vi "Implement Authenticate.vi"(8 "error in (no error)":errorcluster, 10 "Challenge Dict":string, 11 "WampScramAuthenticator in":refnum<class "WampScramAuthenticator.lvclass">) -> (0 "error out":errorcluster, 1 "Authenticate Dict":string, 2 "Authenticate Signature":string, 3 "WampScramAuthenticator out":refnum<class "WampScramAuthenticator.lvclass">)   [LabVIEW 2020, in "wamplv.lvlib" / "WampScramAuthenticator.lvclass"]
uses:
  WampScramAuthenticator.lvclass
  TypeDefs/Authenticate Extra data.ctl
  efa46892-2042-4062-853f-90a4d9cfa7e0.vi
  1957a34c-6116-4582-936f-7ec411d64d2c.vi
  32660840-3418-4907-9075-9fb4615483c7.vi
  <vilib>/JDP Science/JSONtext/Variant to JSON Text.vi
  <vilib>/JDP Science/JSONtext/Set Item.vi
  <vilib>/JDP Science/JSONtext/LVClass Serializer/JSONtext LVClass Serializer.lvclass
  WampScramAuthenticator.lvclass/WampScramAuthenticator.ctl
  Utils/Utils.lvclass
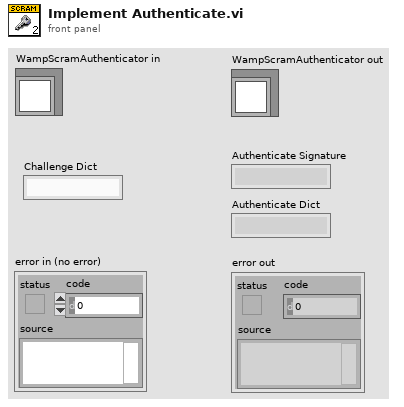
[diagram p1: front panel]
types:
  T1 = typedef "wamplv.lvlib/WampScramAuthenticator.lvclass/Challenge data.ctl" = cluster{"Nonce":string, "kdf":string, "HMAC parameters":T2}
  T2 = typedef "wamplv.lvlib/WampScramAuthenticator.lvclass/HMAC parameters.ctl" = cluster{"Salt":string, "Iterations":i32}
  T3 = typedef "wamplv.lvlib/WampScramAuthenticator.lvclass/Authenticate Extra data.ctl" = cluster{"Nonce":string, "channel_binding":string, "cbind_data":string}
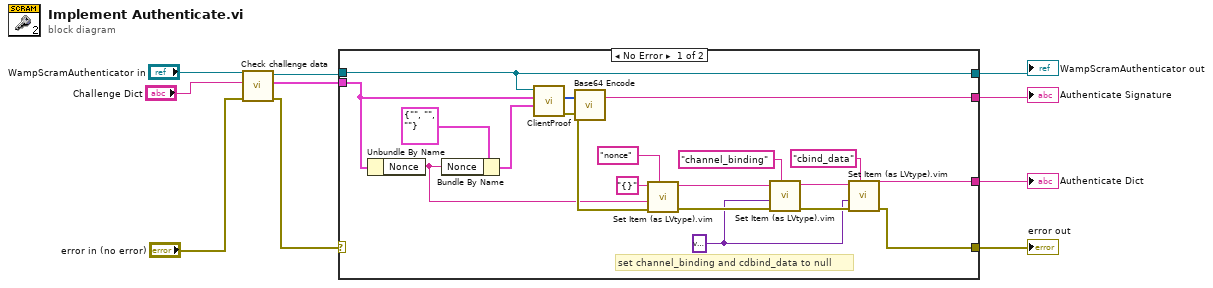
[diagram p0: block diagram]
diagram:
  n1 = call "Check challenge data.vi"("error in (no error)"="error in (no error)", "Challenge Dict"="Challenge Dict", "WampScramAuthenticator in"="WampScramAuthenticator in") -> ("error out"=w4:errorcluster, "Challene data"=w3:T1, "WampScramAuthenticator out"=w5:refnum<class "WampScramAuthenticator.lvclass">)  [unwired: 6 in]
  n2 = case shown="No Error" w4 {
    selector: w4 -> [_ w30]
    tunnel: w5 -> [w28 w31]
    tunnel: [w28 w31] -> w10
    tunnel: [w14 w30] -> w9
    tunnel: w3 -> [w27 _]
    tunnel: [w23 _] -> w2
    tunnel: [w12 _] -> w1
    frame No Error {
      w15 = variant
      # "set channel_binding and cdbind_data to null"
      n3 = Unbundle By Name(w27) -> ("Nonce"=w11:string)
      n4 = Bundle By Name(cluster=T3 {"Nonce"="", "channel_binding"="", "cbind_data"=""} ("Authenticate Extra Data"), "Nonce"=w11) -> (w22:T3)
      n5 = call "ClientProof.vi"("Authenticate Extra  Data"=w22, "Challenge data"=w27, "WampScramAuthenticator in"=w28) -> ("error out"=w13:errorcluster, "ClientProof"=w26:u8[])  [unwired: 6 in, 1 out]
      n6 = call "Base64 Encode.vi"("Bytes"=w26) -> ("Base64 sring out"=w23:string)  [unwired: 2 in]
      n7 = call "Set Item (as LVtype).vim"("$Path or Item Name"="nonce", "error in (no error)"=w13, "Anything"=w11, "JSON"="{}") -> ("error out"=w20:errorcluster, "<JSON>"=w21:string)  [unwired: 4 in, 1 out]
      n8 = call "Set Item (as LVtype).vim"("$Path or Item Name"="channel_binding", "error in (no error)"=w20, "Anything"=w15, "JSON"=w21) -> ("error out"=w17:errorcluster, "<JSON>"=w18:string)  [unwired: 4 in, 1 out]
      n9 = call "Set Item (as LVtype).vim"("$Path or Item Name"="cbind_data", "error in (no error)"=w17, "Anything"=w15, "JSON"=w18) -> ("error out"=w14:errorcluster, "<JSON>"=w12:string)  [unwired: 4 in, 1 out]
    }
    frame Error {
    }
  }
  "error out" <- w9
  "WampScramAuthenticator out" <- w10
  "Authenticate Signature" <- w2
  "Authenticate Dict" <- w1
